vi "Get Foreign Key.vi"(8 "error in (no error)":errorcluster, 9 "Column Name Array":string[](array[string]), 10 "Table Name":string, 11 "Database in":refnum<class "Database.lvclass">) -> (0 "error out":errorcluster, 2 "FK Properties Array":T1[](array[typedef]), 3 "Database out":refnum<class "Database.lvclass">)   [LabVIEW 2020, in "Database.lvclass"]
uses:
  Database.lvclass
  foreign key properties.ctl
  Database Interfaces.lvlib
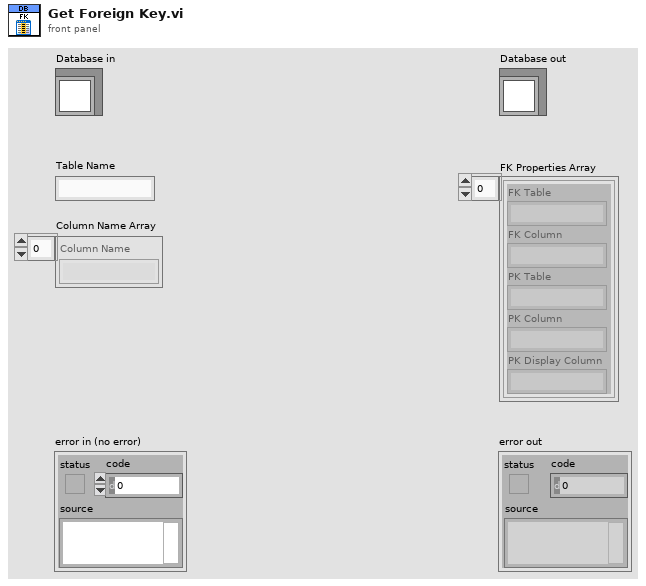
[diagram p1: front panel]
types:
  T1 = typedef "Database Interfaces.lvlib/foreign key properties.ctl" = cluster{"FK Table":string, "FK Column":string, "PK Table":string, "PK Column":string, "PK Display Column":string}
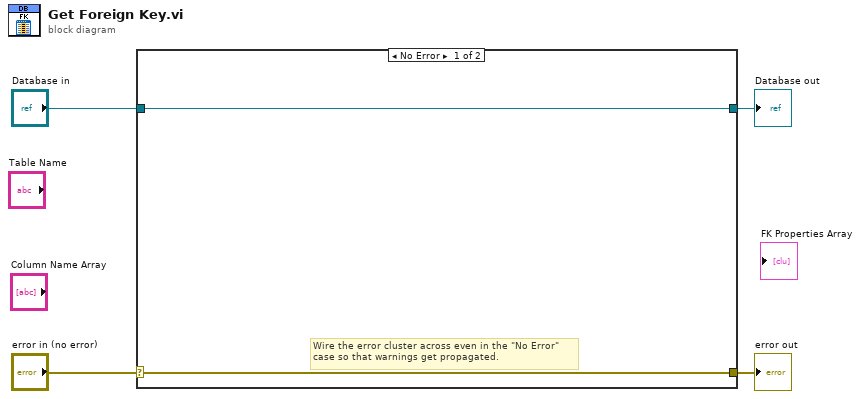
[diagram p0: block diagram]
diagram:
  n1 = case shown="No Error" "error in (no error)" {
    selector: "error in (no error)" -> [w5 w8]
    tunnel: [w5 w8] -> w3
    tunnel: [w6 w7] -> w1
    tunnel: "Database in" -> [w6 w7]
    frame No Error {
      # "Wire the error cluster across even in the \"No Error\"\ncase so that warnings get propagated."
    }
    frame Error {
    }
  }
  "error out" <- w3
  "Database out" <- w1
